vi "Unlock.vi"(11 "UniqueName in":refnum<class "UniqueName.lvclass">) -> (3 "UniqueName out":refnum<class "UniqueName.lvclass">)   [LabVIEW 2014, in "UniqueName.lvlib" / "UniqueName.lvclass"]
uses:
  UniqueName.lvclass
  Command.ctl
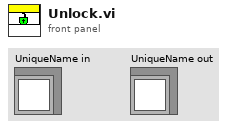
[diagram p1: front panel]
types:
  T1 = typedef "UniqueName.lvlib/UniqueName.lvclass/Command.ctl" = enum16{"Get", "Get All", "Set", "Delete", "Get Status", "Init", "Reserve Ownership", "Release Ownership", "Lock", "Unlock"}
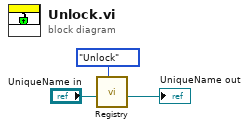
[diagram p0: block diagram]
diagram:
  n1 = call "Registry.vi"("Command (Get)"=Command."Unlock", "UniqueName Object (Set)"="UniqueName in") -> ("Returned Object"=→"UniqueName out":refnum<class "UniqueName.lvclass">)  [unwired: 5 in, 4 out]
